vi "FGen_PXI.vi"(4 "Np":i32, 6 "Ns":i32, 7 "FGen Amplitude (V)":dbl=0.001 format="%#.4f", 8 "error in (no error)":errorcluster, 9 "fp (wfm)":dbl=10000.0 format="%.10f", 10 "fs (input)":dbl, 11 "Instrument Handle":refnum<k15>) -> (0 "error out":errorcluster, 3 "Instrument Handle Out":refnum<k15>)   [LabVIEW 2018]
uses:
  <instrlib>/niFgen/niFgen.llb/niFgen_ctl Sample Clock Source Values (Ring).ctl
  <instrlib>/niFgen/niFgen.llb/niFgen_ctl Exported Signal Name Values (Ring).ctl
  <instrlib>/niFgen/niFgen.llb/niFgen_ctl Exported Signal Identifiers (Ring).ctl
  <instrlib>/niFgen/niFgen.llb/niFgen_ctl Exported Signal Desination Values (ComboBox).ctl
  <instrlib>/niFgen/niFgen.llb/niFgen Create Waveform (WDT).vi
  <vilib>/measure/NI_MABase.lvlib
panel:
  in  "Source (Onboard Clock)":T1="OnboardClock"
  out "Ns (FGen)":dbl=1000.0
  out "fs (output)":dbl=1000.0
  out "Perturbation Waveform":waveform(dbl)(graph)
  in  "Channel":string="0" caption="Channel Name"
  in  "Clock Mode":u32(ring)=1 items=["Hi Resolution Sampling", "Divide Down Sampling"]
  # "Output"
  # "Input (main VI)"
  # "Input (sub VI)"
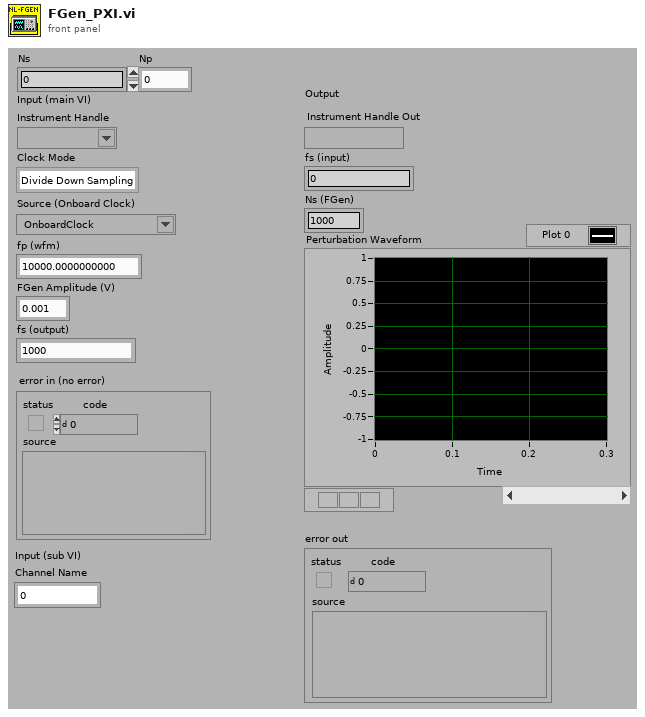
[diagram p1: front panel]
types:
  T1 = typedef "niFgen_ctl Sample Clock Source Values (Ring).ctl" = string
  T2 = typedef "niFgen_ctl Exported Signal Desination Values (ComboBox).ctl" = string
  T3 = typedef "niFgen_ctl Exported Signal Identifiers (Ring).ctl" = string
  T4 = typedef "niFgen_ctl Exported Signal Name Values (Ring).ctl" = u16
  T5 = enum16{"Sine Wave", "Triangle Wave", "Square Wave", "Sawtooth Wave"}
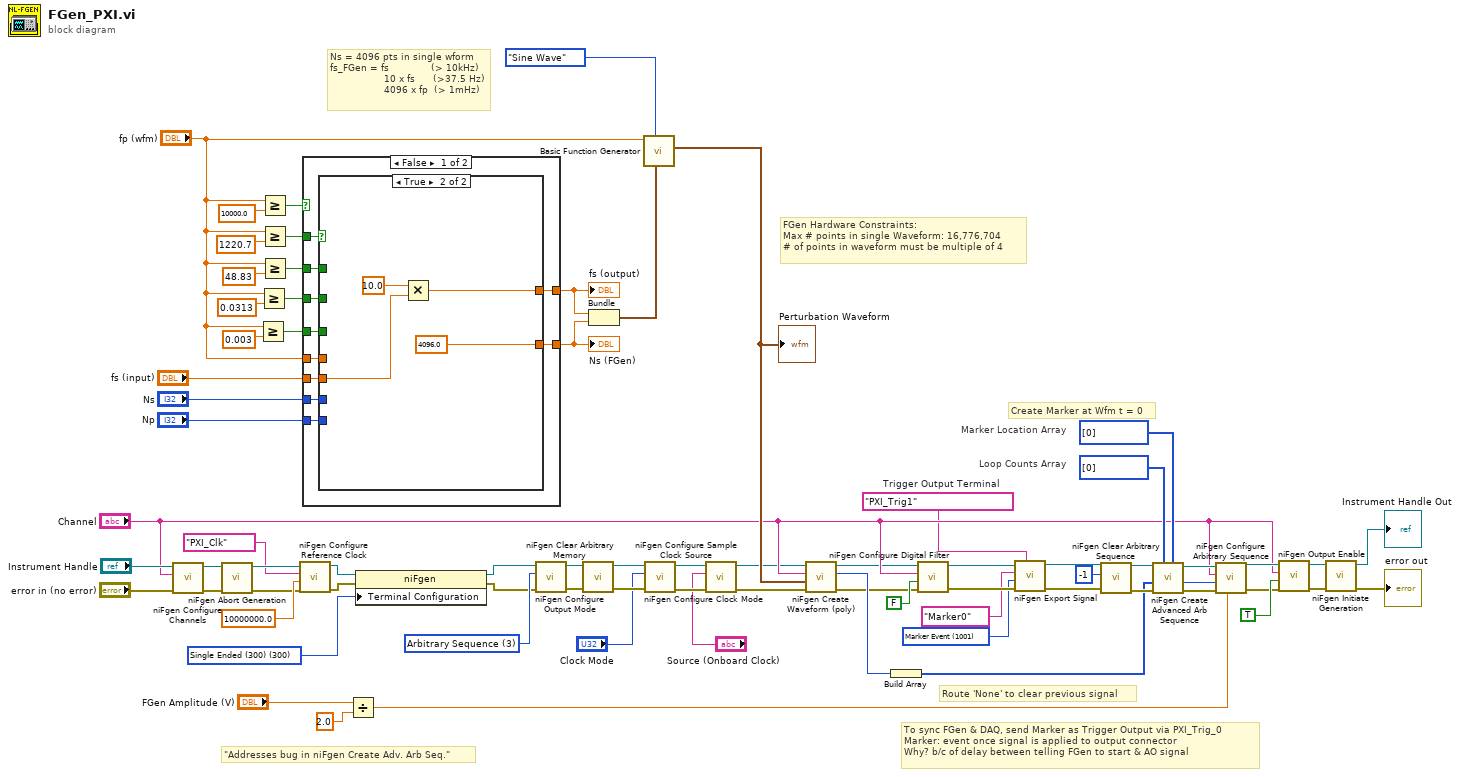
[diagram p0: block diagram]
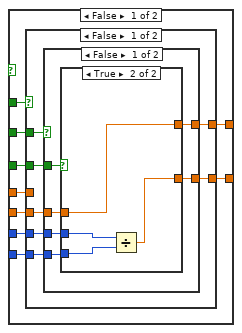
[diagram p2: hidden frame]
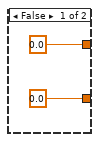
[diagram p3: hidden frame]
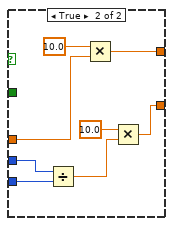
[diagram p4: hidden frame]
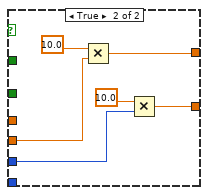
[diagram p5: hidden frame]
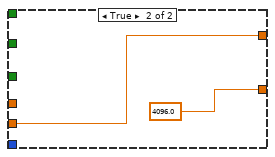
[diagram p6: hidden frame]
diagram:
  w1 = T2 "PXI_Trig1"  # Trigger Output Terminal
  w29 = T4 1001 items=["Sample Clock"=101, "Sample Clock Timebase"=1006, "Reference Clock"=102, "Onboard Reference Clock"=1019, "Start Trigger"=1004, "Script Trigger"=103, "Marker Event"=1001, "Data Marker Event"=108, "Ready For Start Event"=105, "Started Event"=106, "Done Event"=107, "Synchronization Pulse"=1007, "Sync Out"=1002] ("Signal")
  w34 = 300 items=["Single Ended (300)"=300, "Differential (301)"=301] ("Output:Terminal Configuration")
  w72 = u32 3 items=["Standard Function", "Frequency List", "Arbitrary Waveform", "Arbitrary Sequence", "Script"] ("Output Mode")
  # "Create Marker at Wfm t = 0"
  # "To sync FGen & DAQ, send Marker as Trigger Output via PXI_Trig_0\nMarker: event once signal is applied to output connector\nWhy? b/c of delay between telling FGen to start & AO signal"
  # "Ns = 4096 pts in single wform\nfs_FGen = fs              (> 10kHz)\n                  10 x fs      (>37.5 Hz)\n                  4096 x fp  (> 1mHz)"
  # "FGen Hardware Constraints:\nMax # points in single Waveform: 16,776,704\n# of points in waveform must be multiple of 4"
  # "Route 'None' to clear previous signal"
  # "\"Addresses bug in niFgen Create Adv. Arb Seq.\""
  # "Loop Counts Array"
  # "Marker Location Array"
  n1 = call <instrlib>:"niFgen Configure Channels.vi"("error in (no error)"="error in (no error)", "Channels"="Channel", "Instrument Handle"="Instrument Handle") -> ("error out"=w14:errorcluster, "Instrument Handle Out"=w15:refnum<k15>)  [unwired: 7 in]
  n2 = call <instrlib>:"niFgen Abort Generation.vi"("error in (no error)"=w14, "Instrument Handle"=w15) -> ("error out"=w13:errorcluster, "Instrument Handle Out"=w12:refnum<k15>)  [unwired: 8 in]
  n3 = Greater Or Equal?(x="fp (wfm)", y=0.003) -> (x >= y?=w22:bool)
  n4 = Greater Or Equal?(x="fp (wfm)", y=0.0313) -> (x >= y?=w23:bool)
  n5 = Greater Or Equal?(x="fp (wfm)", y=10000.0) -> (x >= y?=w44:bool)
  n6 = Greater Or Equal?(x="fp (wfm)", y=1220.7) -> (x >= y?=w37:bool)
  n7 = Greater Or Equal?(x="fp (wfm)", y=48.83) -> (x >= y?=w45:bool)
  n8 = call <instrlib>:"niFgen Configure Reference Clock.vi"("error in (no error)"=w13, "Reference Clock Frequency"=10000000.0, "Source"="PXI_Clk", "Instrument Handle"=w12) -> ("error out"=w19:errorcluster, "Instrument Handle Out"=w20:refnum<k15>)  [unwired: 6 in]
  n9 = case shown="False" w44 {
    tunnel: [w82 w131] -> w41
    tunnel: [w83 4096.0 ("Fs")] -> w40
    tunnel: w45 -> [w84 _]
    tunnel: "fs (input)" -> [w81 w131]
    tunnel: w37 -> [w80 _]
    tunnel: "fp (wfm)" -> [w79 _]
    tunnel: "Ns" -> [w78 _]
    tunnel: w23 -> [w77 _]
    tunnel: w22 -> [w76 _]
    tunnel: "Np" -> [w75 _]
    frame False {
      n10 = case shown="True" w80 {
        tunnel: w84 -> [w92 _]
        tunnel: [w90 4096.0 ("Fs")] -> w83
        tunnel: [w91 w127] -> w82
        tunnel: w81 -> [w93 w129]
        tunnel: w79 -> [w89 _]
        tunnel: w78 -> [w88 _]
        tunnel: w77 -> [w87 _]
        tunnel: w76 -> [w86 _]
        tunnel: w75 -> [w85 _]
        frame False {
          n11 = case shown="False" w92 {
            tunnel: [w97 w125] -> w91
            tunnel: [w96 w121] -> w90
            tunnel: w93 -> [w98 w124]
            tunnel: w89 -> [_ _]
            tunnel: w88 -> [w95 w122]
            tunnel: w87 -> [w100 _]
            tunnel: w86 -> [w99 _]
            tunnel: w85 -> [w94 _]
            frame False {
              n12 = case shown="False" w100 {
                tunnel: w99 -> [w106 _]
                tunnel: w98 -> [w103 w119]
                tunnel: [w105 w118] -> w97
                tunnel: [w104 w113] -> w96
                tunnel: w95 -> [w102 w117]
                tunnel: w94 -> [w101 w116]
                frame False {
                  n13 = case shown="True" w106 {
                    tunnel: [0.0 ("y") w112] -> w105
                    tunnel: [0.0 ("y") w109] -> w104
                    tunnel: w103 -> [_ w112]
                    tunnel: w102 -> [_ w111]
                    tunnel: w101 -> [_ w110]
                    frame False {
                    }
                    frame True {
                      n14 = Divide(x=w111, y=w110) -> (x/y=w109:dbl)
                    }
                  }
                }
                frame True {
                  n15 = Divide(x=w117, y=w116) -> (x/y=w114:dbl)
                  n16 = Multiply(x=10.0, y=w119) -> (x*y=w118:dbl)
                  n17 = Multiply(x=10.0, y=w114) -> (x*y=w113:dbl)
                }
              }
            }
            frame True {
              n18 = Multiply(x=10.0, y=w124) -> (x*y=w125:dbl)
              n19 = Multiply(x=10.0, y=w122) -> (x*y=w121:dbl)
            }
          }
        }
        frame True {
          n20 = Multiply(x=10.0, y=w129) -> (x*y=w127:dbl)
        }
      }
    }
    frame True {
    }
  }
  "fs (output)" <- w41
  "Ns (FGen)" <- w40
  n21 = Divide(x="FGen Amplitude (V)", y=2.0) -> (x/y=w46:dbl)
  n22 = property class="niFgen"(reference=w20, error in=w19, "Terminal Configuration"=w34) -> (reference out=w11:refnum<k15>, error out=w10:errorcluster)
  n23 = call <instrlib>:"niFgen Configure Output Mode.vi"("error in (no error)"=w10, "Output Mode (default: 0=Standard Function)"=w72, "Instrument Handle"=w11) -> ("error out"=w68:errorcluster, "Instrument Handle Out"=w71:refnum<k15>)  [unwired: 6 in]
  n24 = call <instrlib>:"niFgen Clear Arbitrary Memory.vi"("error in (no error)"=w68, "Instrument Handle"=w71) -> ("error out"=w69:errorcluster, "Instrument Handle Out"=w70:refnum<k15>)  [unwired: 8 in]
  n25 = Bundle("fs (input)"=w41, "Fs"=w40) -> (w50:cluster{"fs (input)":dbl, "Fs":dbl})  [unwired: 1 in]
  n26 = call <vilib>:"Basic Function Generator.vi"("sampling info"=w50, "signal type"=T5."Sine Wave" ("Signal Type"), "frequency"="fp (wfm)") -> ("signal out"=w54:waveform(dbl))  [unwired: 6 in, 2 out]
  "Perturbation Waveform" <- w54
  n27 = call <instrlib>:"niFgen Configure Clock Mode.vi"("error in (no error)"=w69, "Clock Mode (default: 1=divide down)"="Clock Mode", "Instrument Handle"=w70) -> ("error out"=w5:errorcluster, "Instrument Handle Out"=w7:refnum<k15>)  [unwired: 7 in]
  n28 = call <instrlib>:"niFgen Configure Sample Clock Source.vi"("error in (no error)"=w5, "Source (Onboard Clock)"="Source (Onboard Clock)", "Instrument Handle"=w7) -> ("error out"=w4:errorcluster, "Instrument Handle Out"=w6:refnum<k15>)  [unwired: 7 in]
  n29 = call-poly <instrlib>:"niFgen Create Waveform (poly).vi"("error in (no error)"=w4, "Waveform"=w54, "Channel Name"="Channel", "Instrument Handle"=w6) -> ("error out"=w8:errorcluster, "Waveform Handle"=w53:i32, "Instrument Handle Out"=w9:refnum<k15>)  [unwired: 5 in]
  n30 = Build Array "Build Array"(w53) -> (w61:i32[])
  n31 = call <instrlib>:"niFgen Configure Digital Filter.vi"("error in (no error)"=w8, "Digital Filter Enable (default: True)"=FALSE, "Channel Name"="Channel", "Instrument Handle"=w9) -> ("error out"=w32:errorcluster, "Instrument Handle Out"=w33:refnum<k15>)  [unwired: 6 in]
  n32 = call <instrlib>:"niFgen Export Signal.vi"("Output Terminal (do not export)"=w1, "error in (no error)"=w32, "Signal"=w29, "Signal Identifier (None)"=T3 "Marker0", "Instrument Handle"=w33) -> ("error out"=w30:errorcluster, "Instrument Handle Out"=w31:refnum<k15>)  [unwired: 5 in]
  n33 = call <instrlib>:"niFgen Clear Arbitrary Sequence.vi"("error in (no error)"=w30, "Sequence Handle"=-1 ("sequence handle"), "Instrument Handle"=w31) -> ("error out"=w64:errorcluster, "Instrument Handle Out"=w65:refnum<k15>)  [unwired: 7 in]
  n34 = call <instrlib>:"niFgen Create Advanced Arb Sequence.vi"("Marker Location Array"=i32[] [0] ("loop counts array"), "Loop Counts Array"=i32[] [0] ("loop counts array"), "error in (no error)"=w64, "Waveform Handles Array"=w61, "Instrument Handle"=w65) -> ("error out"=w59:errorcluster, "Sequence Handle"=w56:i32, "Instrument Handle Out"=w60:refnum<k15>)  [unwired: 3 in, 1 out]
  n35 = call <instrlib>:"niFgen Configure Arbitrary Sequence.vi"("Gain"=w46, "error in (no error)"=w59, "Sequence Handle"=w56, "Channel Name"="Channel", "Instrument Handle"=w60) -> ("error out"=w58:errorcluster, "Instrument Handle Out"=w57:refnum<k15>)  [unwired: 5 in]
  n36 = call <instrlib>:"niFgen Output Enable.vi"("error in (no error)"=w58, "Output Enable (default: True)"=TRUE ("output enable"), "Channel Name"="Channel", "Instrument Handle"=w57) -> ("error out"=w73:errorcluster, "Instrument Handle Out"=w74:refnum<k15>)  [unwired: 6 in]
  n37 = call <instrlib>:"niFgen Initiate Generation.vi"("error in (no error)"=w73, "Instrument Handle"=w74) -> ("error out"=→"error out":errorcluster, "Instrument Handle Out"=→"Instrument Handle Out":refnum<k15>)  [unwired: 8 in]
